vi "prepareStreamingDataAlgorithm.vi"(8 "error in (no error)":errorcluster, 10 "Stream Mode Algorithm":T1, 11 "Model in":refnum<class "Model.lvclass">) -> (0 "error out":errorcluster, 3 "Model out":refnum<class "Model.lvclass">)   [LabVIEW 2013, in "Model.lvclass"]
uses:
  Model.lvclass
  Configuration/Stream Mode Algorithm.ctl
  Model.lvclass/Model.ctl
  ISDAFactory/ISDAFactory.lvclass
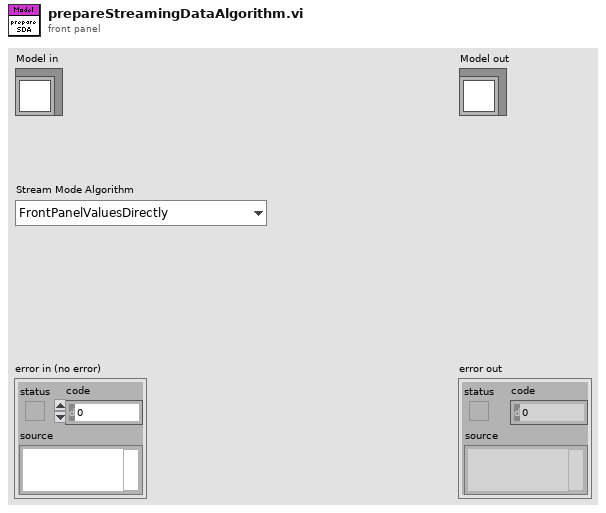
[diagram p1: front panel]
types:
  T1 = typedef "Stream Mode Algorithm.ctl" = enum16{"FrontPanelValuesDirectly"}
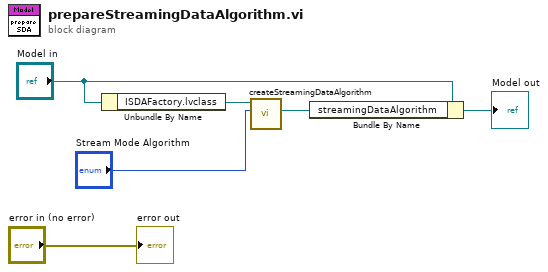
[diagram p0: block diagram]
diagram:
  n1 = Unbundle By Name("Model in") -> ("ISDAFactory.lvclass"=w3:refnum<class "ISDAFactory.lvclass">)
  n2 = call-dynamic "createStreamingDataAlgorithm.vi"("Stream Mode Algorithm"="Stream Mode Algorithm", "ISDAFactory in"=w3) -> ("StreamingDataAlgorithm"=w1:refnum<class "StreamingDataAlgorithm.lvclass">)  [unwired: 7 in, 2 out]
  n3 = Bundle By Name(cluster="Model in", "streamingDataAlgorithm"=w1) -> (→"Model out":refnum<class "Model.lvclass">)
  "error out" <- "error in (no error)"
